vi "readFile.vi"(7 "New (one file)":bool=TRUE, 8 "error in (no error)":errorcluster, 11 "Cam 1":T2) -> (0 "error out":errorcluster, 2 "Cluster":T1, 3 "Cam 0":T2)   [LabVIEW 2013]
uses:
  CamSettingSUB_TypDEf.ctl
  support0/CamAndObj_TypDEf.ctl
  OnOffTypeDef.ctl
  userROI.ctl
  source/Device Driver/shared/numericVariable_TypeDef.ctl
  CamRoiTypDef.ctl
  configTypDEf.ctl
  source/Device Driver/BaseDriver/BaseDriver.lvclass
panel:
  out "all rows":string[][](array[string])
  out "appended array":string[](array[string])
  out "Spec_Calib_file 2":path
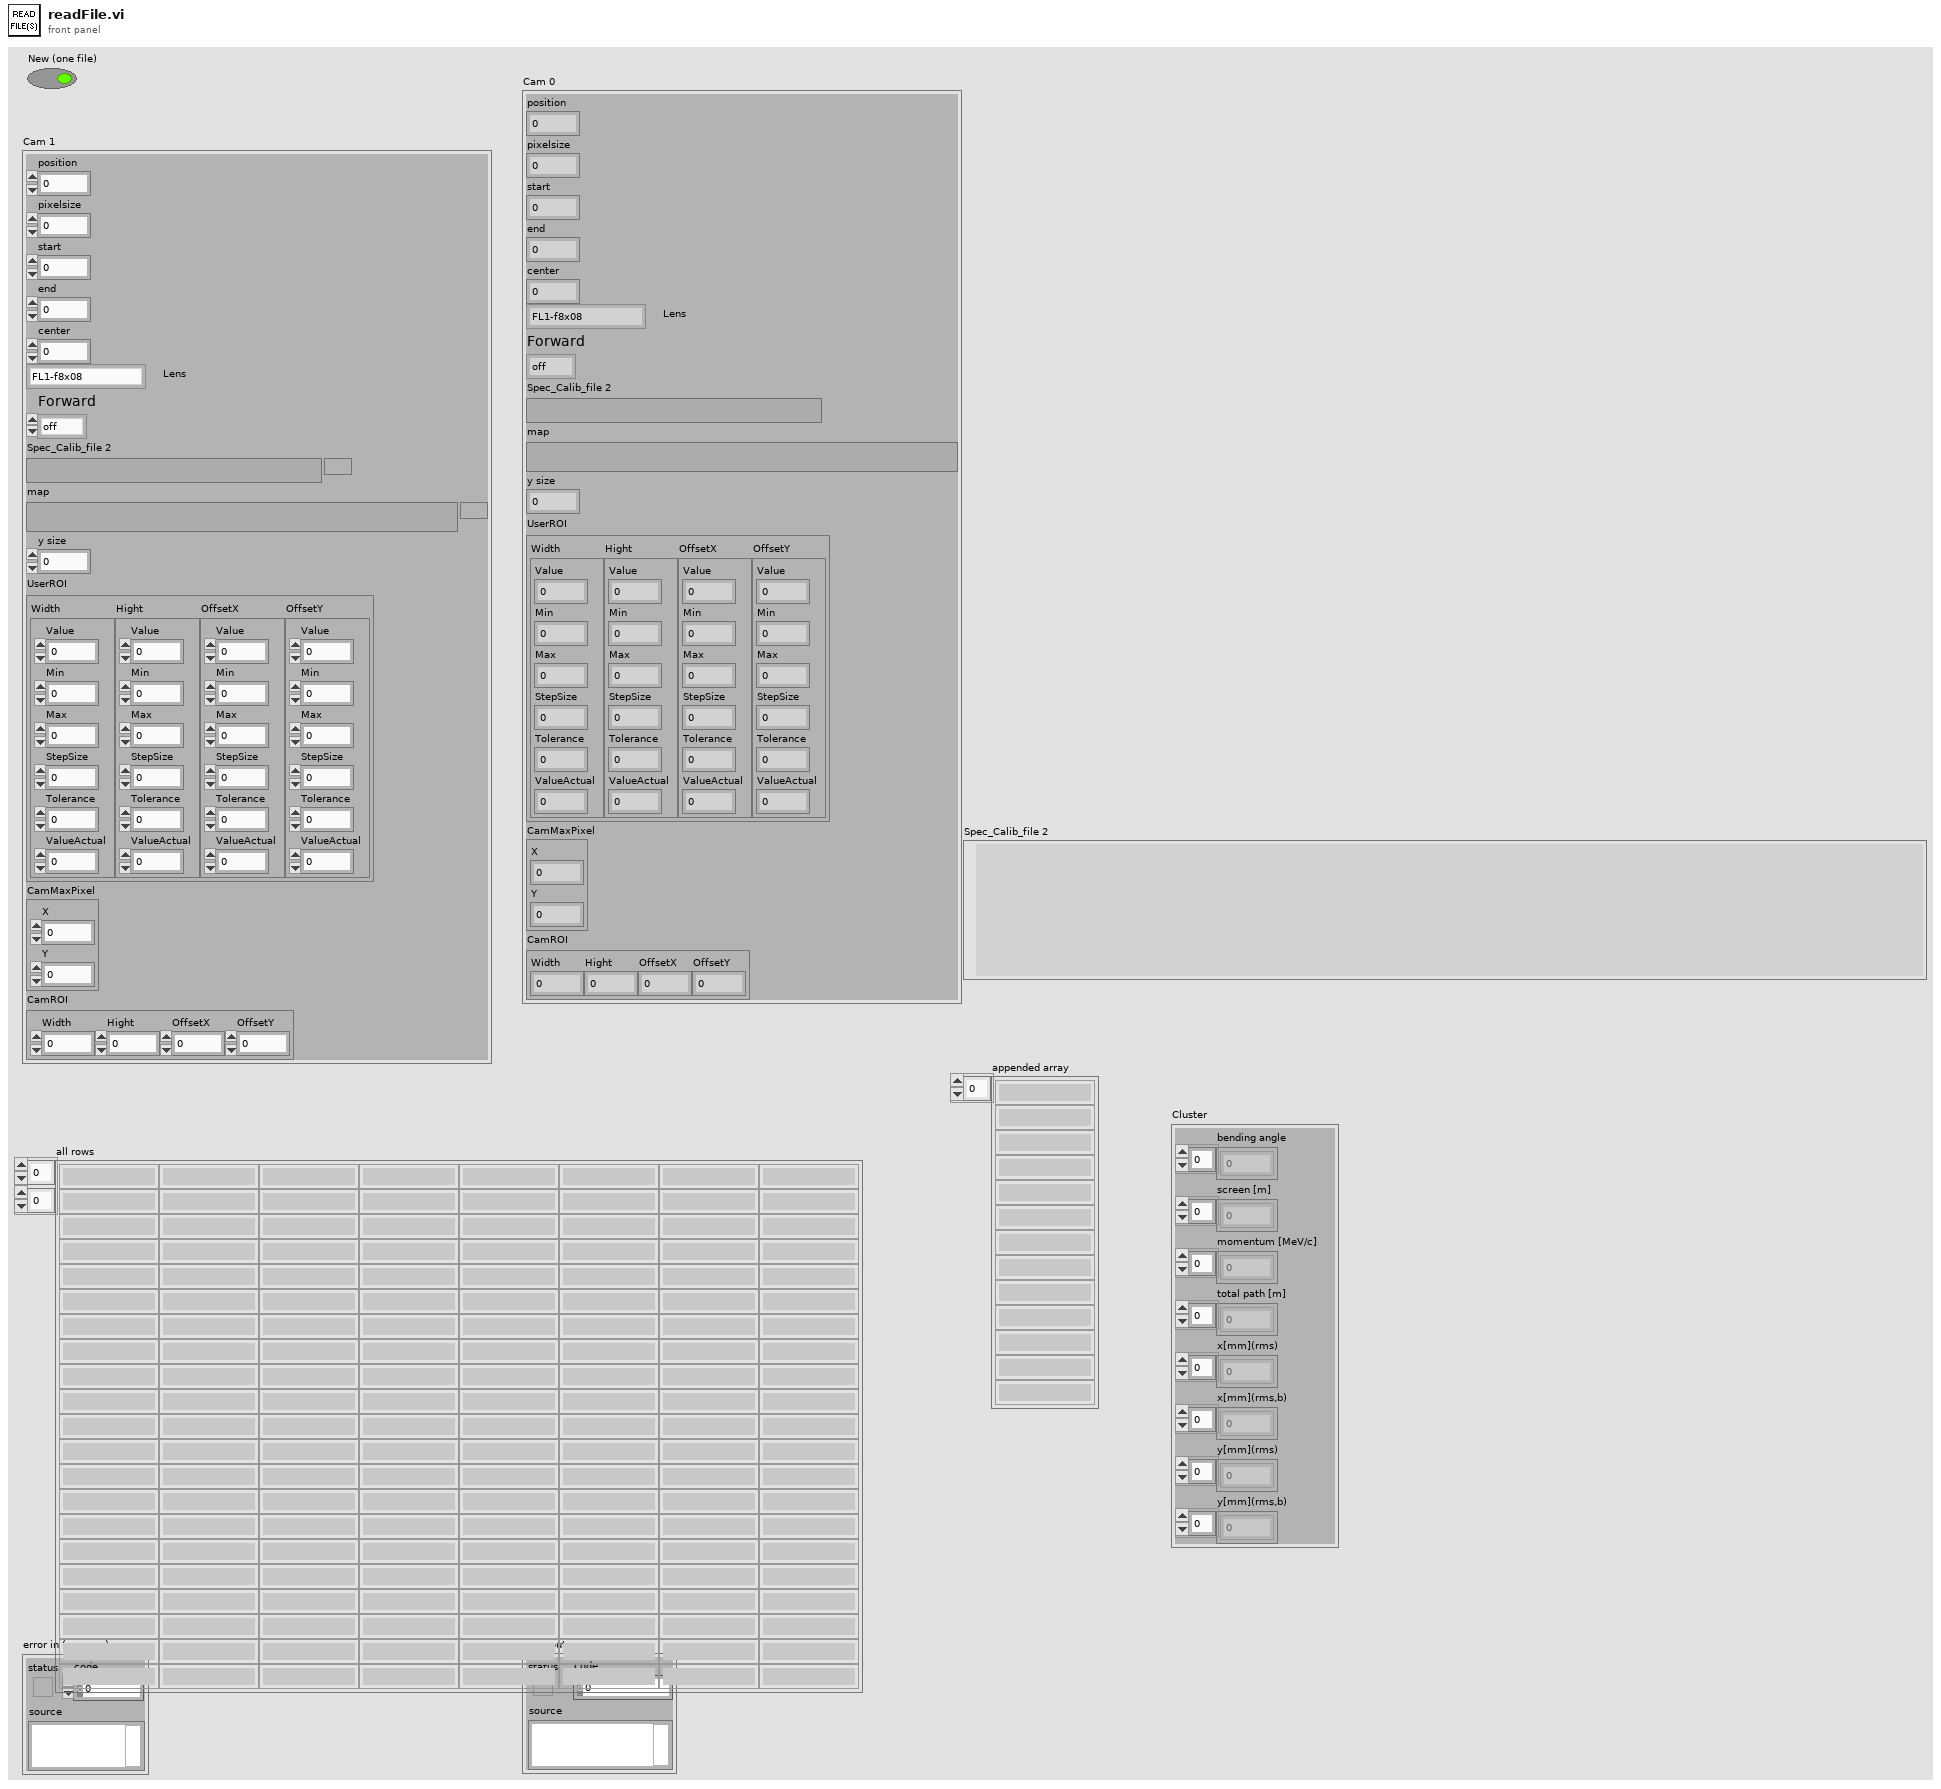
[diagram p1: front panel]
types:
  T1 = typedef "configTypDEf.ctl" = cluster{"bending angle":dbl[], "screen [m]":dbl[], "momentum [MeV/c]":dbl[], "total path [m]":dbl[], "x[mm](rms)":dbl[], "x[mm](rms,b)":dbl[], "y[mm](rms)":dbl[], "y[mm](rms,b)":dbl[]}
  T2 = typedef "CamSettingSUB_TypDEf.ctl" = cluster{"position":dbl, "pixelsize":dbl, "start":dbl, "end":dbl, "center":dbl, "Lens":T3, "Forward":T4, "Spec_Calib_file 2":path, "map":path, "y size":i32, "UserROI":T5, "CamMaxPixel":cluster{"X":i32, "Y":i32}, "CamROI":T7}
  T3 = typedef "CamAndObj_TypDEf.ctl" = enum16{"FL1-f8x08", "FL1-f8x06", "FL1-f8", "ch300-f50", "FL2G-f8", "FL3M14-f8", "FL3M14-f8x08", "FL3M14-f8x08(2x2)"}
  T4 = typedef "OnOffTypeDef.ctl" = enum16{"off", "on"}
  T5 = typedef "userROI.ctl" = cluster{"Width":T6, "Hight":T6, "OffsetX":T6, "OffsetY":T6}
  T6 = typedef "BaseDriver.lvclass/numericVariable_TypeDef.ctl" = cluster{"Value":dbl, "Min":dbl, "Max":dbl, "StepSize":dbl, "Tolerance":dbl, "ValueActual":dbl}
  T7 = typedef "CamRoiTypDef.ctl" = cluster{"Width":dbl, "Hight":dbl, "OffsetX":dbl, "OffsetY":dbl}
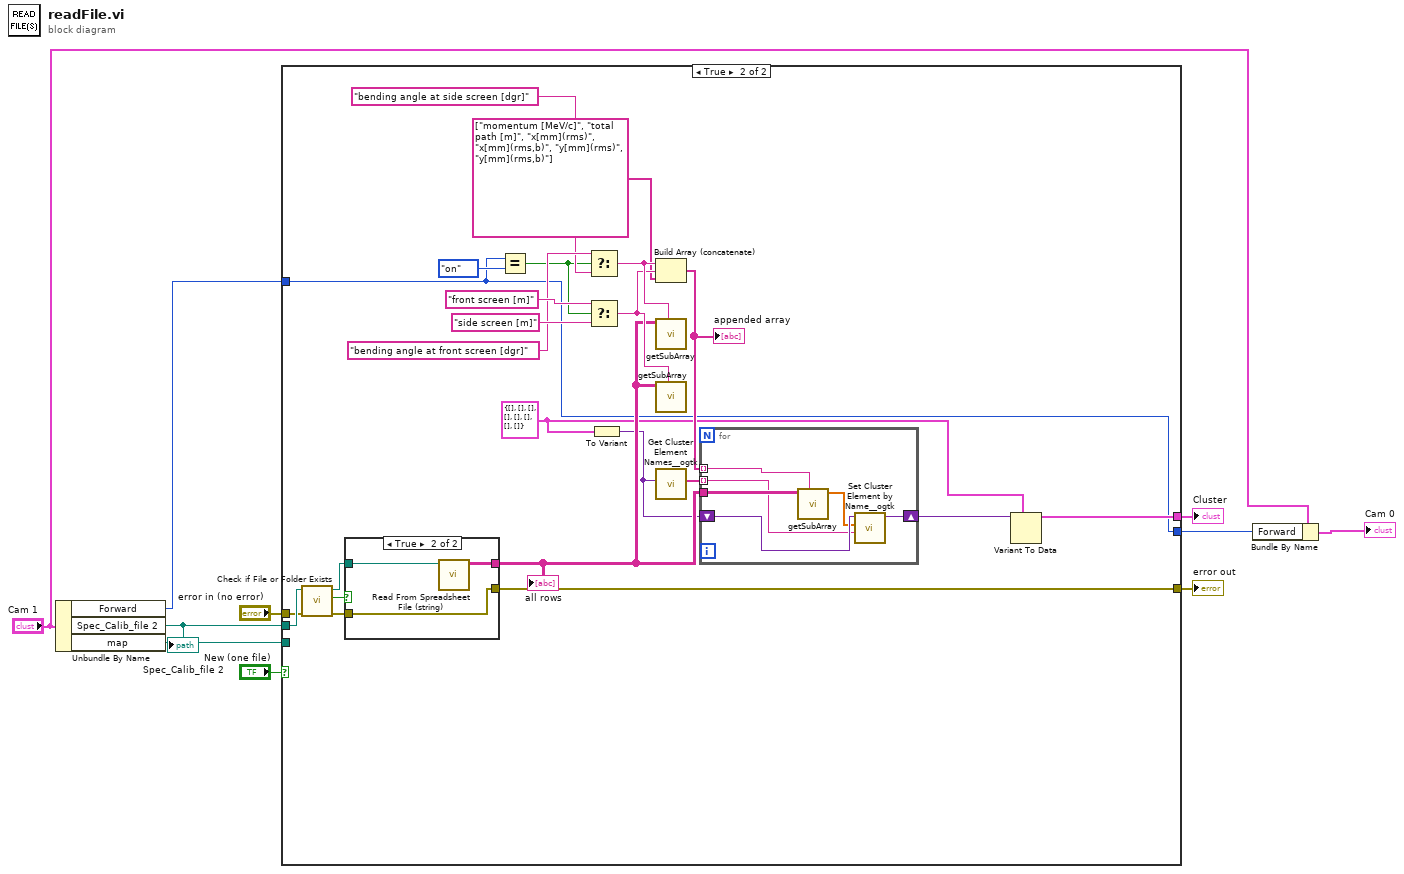
[diagram p0: block diagram]
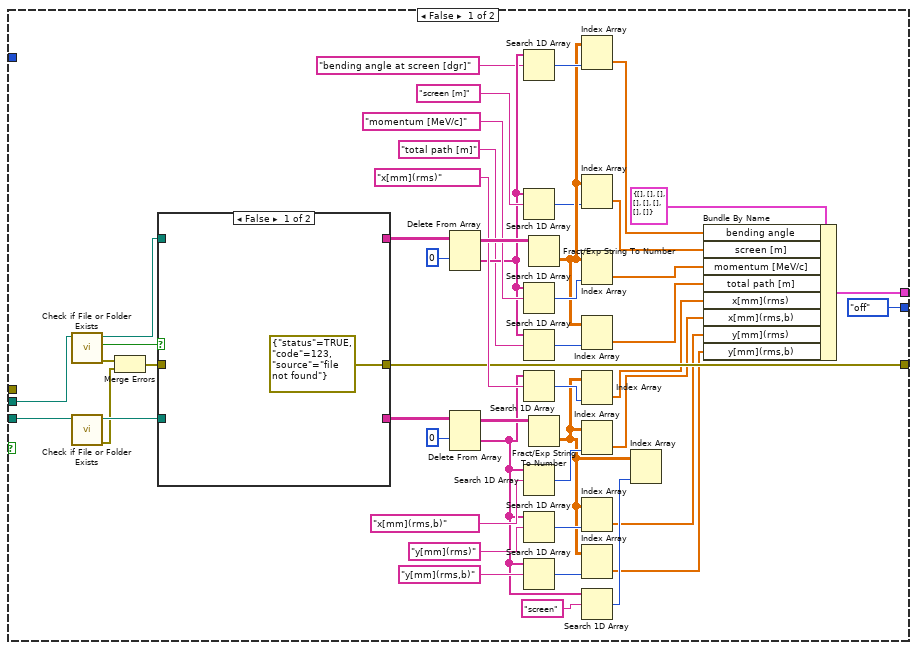
[diagram p2: hidden frame]
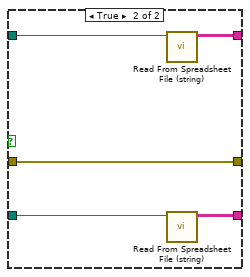
[diagram p3: hidden frame]
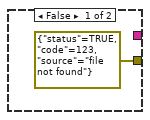
[diagram p4: hidden frame]
diagram:
  n1 = Unbundle By Name("Cam 1") -> ("Forward"=w5:T4, "Spec_Calib_file 2"=w9:path, "map"=w10:path)
  "Spec_Calib_file 2" <- w9
  n2 = case shown="True" "New (one file)" {
    tunnel: w9 -> [w29 w83]
    tunnel: w10 -> [w27 _]
    tunnel: w5 -> [_ w66]
    tunnel: [OnOffTypeDef."off" ("Forward") w66] -> w7
    tunnel: [w22 w79] -> w3
    tunnel: "error in (no error)" -> [_ w81]
    tunnel: [w11 w68] -> w1
    frame False {
      n3 = call "Check if File or Folder Exists.vi"("path"=w29) -> ("error out"=w25:errorcluster, "file or folder exists?"=w23:bool, "dup path"=w28:path)  [unwired: 8 in]
      n4 = call "Check if File or Folder Exists.vi"("path"=w27) -> ("error out"=w24:errorcluster, "dup path"=w26:path)  [unwired: 8 in, 1 out]
      n5 = Merge Errors(w25, w24) -> (w21:errorcluster)
      n6 = case shown="False" w23 {
        tunnel: [_ w64] -> w58
        tunnel: [_ w63] -> w49
        tunnel: w28 -> [_ w62]
        tunnel: w26 -> [_ w61]
        tunnel: [errorcluster {"status"=TRUE, "code"=123, "source"="file not found"} ("error out") w60] -> w22
        tunnel: w21 -> [_ w60]
        frame False {
        }
        frame True {
          n7 = call "Read From Spreadsheet File (string).vi"("file path (dialog if empty)"=w62) -> ("all rows"=w64:string[][])  [unwired: 6 in, 4 out]
          n8 = call "Read From Spreadsheet File (string).vi"("file path (dialog if empty)"=w61) -> ("all rows"=w63:string[][])  [unwired: 6 in, 4 out]
        }
      }
      n9 = Delete From Array(array=w58, index (row)=0) -> (deleted portion=w37:string[], array with subset deleted=w56:string[][])  [unwired: 2 in]
      n10 = Delete From Array(array=w49, index (row)=0) -> (deleted portion=w38:string[], array with subset deleted=w51:string[][])  [unwired: 2 in]
      n11 = Search 1D Array(1D array=w37, element="bending angle at screen [dgr]") -> (index of element=w54:i32)  [unwired: 1 in]
      n12 = Search 1D Array(1D array=w37, element="screen [m]") -> (index of element=w32:i32)  [unwired: 1 in]
      n13 = Search 1D Array(1D array=w37, element="momentum [MeV/c]") -> (index of element=w52:i32)  [unwired: 1 in]
      n14 = Search 1D Array(1D array=w37, element="total path [m]") -> (index of element=w34:i32)  [unwired: 1 in]
      n15 = Search 1D Array(1D array=w38, element="x[mm](rms)") -> (index of element=w47:i32)  [unwired: 1 in]
      n16 = Search 1D Array(1D array=w38, element="x[mm](rms,b)") -> (index of element=w46:i32)  [unwired: 1 in]
      n17 = Search 1D Array(1D array=w38, element="y[mm](rms)") -> (index of element=w45:i32)  [unwired: 1 in]
      n18 = Search 1D Array(1D array=w38, element="y[mm](rms,b)") -> (index of element=w42:i32)  [unwired: 1 in]
      n19 = Fract/Exp String To Number(string=w56) -> (number=w35:dbl[][])  [unwired: 3 in, 1 out]
      n20 = Fract/Exp String To Number(string=w51) -> (number=w39:dbl[][])  [unwired: 3 in, 1 out]
      n21 = Index Array(array=w35, index (col)=w54) -> (element=w12:dbl[])  [unwired: 1 in]
      n22 = Index Array(array=w35, index (col)=w32) -> (element=w13:dbl[])  [unwired: 1 in]
      n23 = Index Array(array=w35, index (col)=w52) -> (element=w19:dbl[])  [unwired: 1 in]
      n24 = Index Array(array=w35, index (col)=w34) -> (element=w18:dbl[])  [unwired: 1 in]
      n25 = Index Array(array=w39, index (col)=w47) -> (element=w17:dbl[])  [unwired: 1 in]
      n26 = Index Array(array=w39, index (col)=w46) -> (element=w16:dbl[])  [unwired: 1 in]
      n27 = Index Array(array=w39, index (col)=w45) -> (element=w15:dbl[])  [unwired: 1 in]
      n28 = Index Array(array=w39, index (col)=w42) -> (element=w14:dbl[])  [unwired: 1 in]
      n29 = Search 1D Array(1D array=w38, element="screen") -> (index of element=w48:i32)  [unwired: 1 in]
      n30 = Index Array(array=w39, index (col)=w48) -> ()  [unwired: 1 in, 1 out]
      n31 = Bundle By Name(cluster=T1 {"bending angle"=[], "screen [m]"=[], "momentum [MeV/c]"=[], "total path [m]"=[], "x[mm](rms)"=[], "x[mm](rms,b)"=[], "y[mm](rms)"=[], "y[mm](rms,b)"=[]}, "bending angle"=w12, "screen [m]"=w13, "momentum [MeV/c]"=w19, "total path [m]"=w18, "x[mm](rms)"=w17, "x[mm](rms,b)"=w16, "y[mm](rms)"=w15, "y[mm](rms,b)"=w14) -> (w11:T1)
    }
    frame True {
      w71 = T1 {"bending angle"=[], "screen [m]"=[], "momentum [MeV/c]"=[], "total path [m]"=[], "x[mm](rms)"=[], "x[mm](rms,b)"=[], "y[mm](rms)"=[], "y[mm](rms,b)"=[]}
      n32 = call "Check if File or Folder Exists.vi"("error in (no error)"=w81, "path"=w83) -> ("error out"=w78:errorcluster, "file or folder exists?"=w80:bool, "dup path"=w82:path)  [unwired: 7 in]
      n33 = case shown="True" w80 {
        tunnel: [_ w97] -> w73
        tunnel: w82 -> [_ w96]
        tunnel: [errorcluster {"status"=TRUE, "code"=123, "source"="file not found"} ("error out") w95] -> w79
        tunnel: w78 -> [_ w95]
        frame False {
        }
        frame True {
          n34 = call "Read From Spreadsheet File (string).vi"("file path (dialog if empty)"=w96) -> ("all rows"=w97:string[][])  [unwired: 6 in, 4 out]
        }
      }
      "all rows" <- w73
      n35 = Equal?(x=w66, y=OnOffTypeDef."on" ("x")) -> (x = y?=w65:bool)
      n36 = Select(t="bending angle at front screen [dgr]" ("element"), s=w65, f="bending angle at side screen [dgr]" ("element")) -> (s? t:f=w77:string)
      n37 = Select(t="front screen [m]" ("element"), s=w65, f="side screen [m]" ("element")) -> (s? t:f=w76:string)
      n38 = To Variant(anything=w71) -> (Variant=w70:variant)
      n39 = Build Array (concatenate)(w77, w76, string[] ["momentum [MeV/c]", "total path [m]", "x[mm](rms)", "x[mm](rms,b)", "y[mm](rms)", "y[mm](rms,b)"]) -> (w74:string[])
      "appended array" <- w74
      n40 = call "getSubArray.vi"("element"=w77, "all rows 2"=w73) -> ()  [unwired: 9 in, 1 out]
      n41 = call "getSubArray.vi"("element"=w76, "all rows 2"=w73) -> ()  [unwired: 9 in, 1 out]
      n42 = call "Get Cluster Element Names__ogtk.vi"("Cluster"=w70) -> ("Element Names"=w69:string[])  [unwired: 9 in, 1 out]
      n43 = for {
        tunnel: w74 -> [w89] mode=indexing
        tunnel: w73 -> [w93]
        shift-right: [w91] -> w72
        shift-left: w70 -> [w92]
        tunnel: w69 -> [w88] mode=indexing
        n44 = call "getSubArray.vi"("element"=w89, "all rows 2"=w93) -> ("Array out"=w90:dbl[])  [unwired: 9 in]
        n45 = call "Set Cluster Element by Name__ogtk.vi"("Element Name (\"\": New Element Data Name)"=w88, "New Element Value"=w90, "Cluster"=w92) -> ("VCluster out"=w91:variant)  [unwired: 6 in, 2 out]
      }
      n46 = Variant To Data(type=w71, Variant=w72) -> (data=w68:T1)  [unwired: 1 in, 1 out]
    }
  }
  "Cluster" <- w1
  "error out" <- w3
  n47 = Bundle By Name(cluster="Cam 1", "Forward"=w7) -> (→"Cam 0":T2)
